vi "CaLabGet_Main.vi"(0 "PV Name":string[](array[string]), 1 "variable PV names (F)":bool, 7 "Field Names":string[](array[string]), 9 "Timeout (3)":dbl, 11 "error in (no error)":errorcluster, 12 "NoMDEL(F)":bool) -> (4 "PV Name (dup)":string[](array[string]), 6 "1rst Value (string)":string[](array[string]), 8 "1rst Value (number)":dbl[](array[numeric]), 10 "Value Array (number)":dbl[][](array[numeric]), 13 "Status":bool, 14 "PV Info":T1[](array[typedef]), 15 "error out":errorcluster)   [LabVIEW 2018]
doc: "This is a VI for reading values of EPICS variables.\n\nINPUT:\n <b>PV Name</b>\n name array of EPICS variables\n <b>Field Names</b>\n optional\n string array of EPICS fields (\"EGU\", \"DESCRIPTION\" etc.)\n <b>Timeout (3)</b>\n optional\n timeout for Channel Access requests in seconds\n <b>NoMDEL (F)</b>\n optional\n true: ignore monitor dead-band of Channel Access (EPICS)\n <b>variable PV names (F)</b>\n optional\n true: in case of changing PV names at PV name input (performance drop)\n <b>Error in (no error)</b>\n\nOUTPUT:\n <b>PV Name</b>\n name array of EPICS variables\n <b>1st Value(string)</b>\n value of variable as String\n shows first item of value array\n <b>1st Value(number)</b>\n value of variable as Double\n shows first item of value array\n <b>Value Array(number)</b>\n all values of variable in Double array\n <b>Error out</b>\n <b>PV Info</b>\n cluster array of full answer\n value array(number)\n PV name\n elements\n size of value array\n value array(string)\n all values of variable in string array\n value array(number)\n elements\n size of value array\n status(string)\n status of EPICS PV as String\n status(number)\n status of EPICS PV as Long\n severity(string)\n severity of EPICS PV as String\n severity(number)\n severity of EPICS PV as Long\n time stamp(string)\n stamp of EPICS PV time as String\n time stamp(number)\n stamp of EPICS PV as Long\n field names\n field values\n string array of requsted EPICS field values\n error IO\n <b>Status</b>\n FALSE: request successful\n TRUE: warnings or errors"
uses:
  <userlib>/caLab/PV Info.ctl
  <userlib>/caLab/lib/caLab.dll
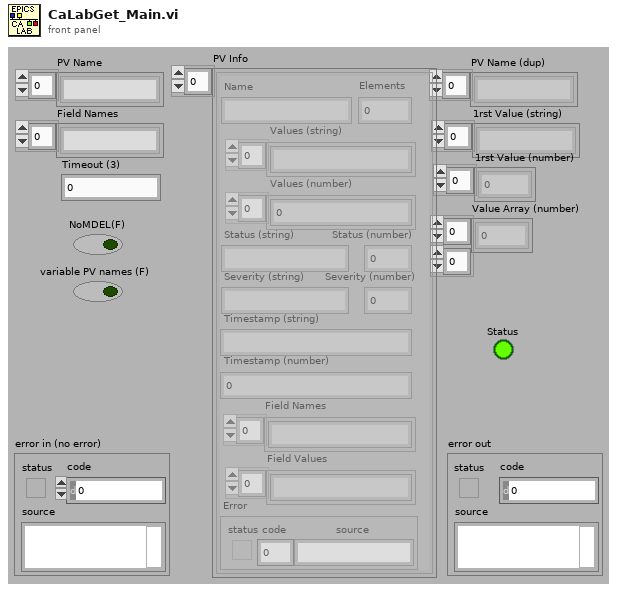
[diagram p1: front panel]
types:
  T1 = typedef "PV Info.ctl" = cluster{"Name":string, "Elements":i32, "Values (string)":string[], "Values (number)":dbl[], "Status (string)":string, "Status (number)":i16, "Severity (string)":string, "Severity (number)":i16, "Timestamp (string)":string, "Timestamp (number)":i32, "Field Names":string[], "Field Values":string[], "Error":errorcluster}
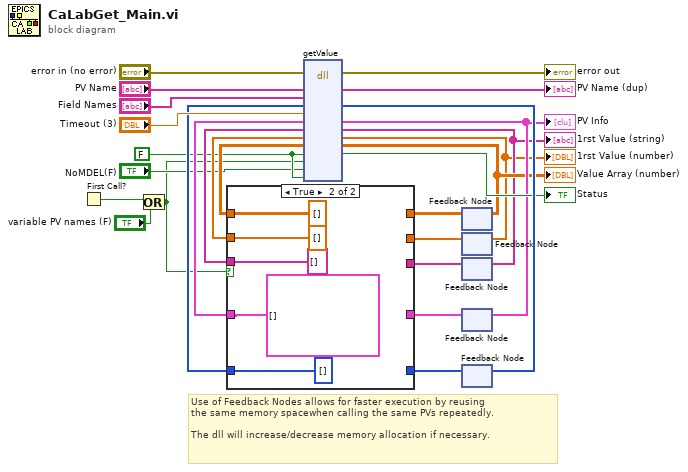
[diagram p0: block diagram]
diagram:
  w5 = FALSE
  # "Use of Feedback Nodes allows for faster execution by reusing\nthe same memory spacewhen calling the same PVs repeatedly.\n\nThe dll will increase/decrease memory allocation if necessary."
  n1 = First Call?() -> (First Call?: T/F=w1:bool)
  n2 = Or(x=w1, y="variable PV names (F)") -> (x .or. y?=w3:bool)
  n3 = feedback #1() -> (w12:dbl[][])  [unwired: 1 out]
  n4 = feedback #2() -> (w10:dbl[])  [unwired: 1 out]
  n5 = feedback #3() -> (w8:string[])  [unwired: 1 out]
  n6 = feedback #4() -> (w22:T1[])  [unwired: 1 out]
  n7 = feedback #5() -> (w21:u64[])  [unwired: 1 out]
  n8 = case shown="True" w3 {
    tunnel: [w32 T1[] [] ("PV Info")] -> w20
    tunnel: [w31 u64[] [] ("value array (number)")] -> w19
    tunnel: w22 -> [w32 _]
    tunnel: w21 -> [w31 _]
    tunnel: [w30 dbl[][] []] -> w14
    tunnel: w12 -> [w30 _]
    tunnel: [w29 dbl[] []] -> w11
    tunnel: w10 -> [w29 _]
    tunnel: [w28 string[] []] -> w9
    tunnel: w8 -> [w28 _]
    frame False {
    }
    frame True {
    }
  }
  n9 = dll-call lib="D:/Program Files (x86)/National Instruments/LabVIEW 2018/user.lib/caLab/lib/calab.dll" fn="getValue" label="caLabGet"(error in="error in (no error)", "PVNameArray"="PV Name", "FieldNameArray"="Field Names", "IndexArray"=w19, "Timeout"="Timeout (3)", "ResultClusterArray"=w20, "FirstStringValue"=w9, "FirstDoubleValue"=w11, "DoubleValueArray"=w14, "status"=w5, "FirstCall"=w3, "NoMDEL"="NoMDEL(F)", "IsInitialized"=w5) -> (error out=→"error out":errorcluster, "PVNameArray"=→"PV Name (dup)":string[], "IndexArray"=w18:u64[], "ResultClusterArray"=w15:T1[], "FirstStringValue"=w7:string[], "FirstDoubleValue"=w6:dbl[], "DoubleValueArray"=w13:dbl[][], "status"=→"Status":bool)  [unwired: 7 in, 2 out]
  "1rst Value (string)" <- w7
  "1rst Value (number)" <- w6
  "Value Array (number)" <- w13
  "PV Info" <- w15
  n10 = feedback-in #1(w13) -> ()
  n11 = feedback-in #2(w6) -> ()
  n12 = feedback-in #3(w7) -> ()
  n13 = feedback-in #4(w15) -> ()
  n14 = feedback-in #5(w18) -> ()
